vi "Proxy.vi"(8 "Globals":refnum<data-value>, 9 "E-Stop":refnum<user-event>, 10 "Response":refnum<user-event>, 11 "RequestMQ":refnum<queue>) -> ()   [LabVIEW 2020, in "Demo.lvlib" / "DemoModule1.lvclass"]
uses:
  DemoModule1.lvclass
  RPC/TypeDefs/Request.ctl
  RPC/TypeDefs/Response.ctl
  RPC.lvlib
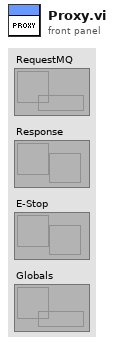
[diagram p1: front panel]
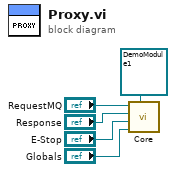
[diagram p0: block diagram]
diagram:
  n1 = call-dynamic "Core.vi"("ObjRef"=refnum<class "DemoModule1.lvclass"> refnum ("Demo.lvlib:DemoModule1.lvclass"), "Globals"="Globals", "E-Stop"="E-Stop", "Response"="Response", "RequestMQ"="RequestMQ") -> ()  [unwired: 7 in]
